vi "RunAsStartupBuzzerTest.vi"() -> ()   [LabVIEW 2020]
uses:
  <vilib>/CISH Robotics/L4VMX VMXpi/Type Def/VMX Channel Index.ctl
  <vilib>/CISH Robotics/L4VMX VMXpi/Digital Output/Digital Output.lvclass
  <vilib>/CISH Robotics/L4VMX VMXpi/L4VMX.lvlib
  <vilib>/CISH Robotics/L4VMX VMXpi/Digital Input/Digital Input.lvclass
panel:
  in  "Stop Button":bool
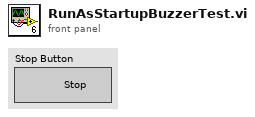
[diagram p1: front panel]
types:
  T1 = typedef "L4VMX.lvlib/VMX Channel Index.ctl" = enum16{"0", "1", "2", "3", "4", "5", "6", "7", "8", "9", "10", "11", "12", "13", "14", "15", "16", "17", "18", "19", "20", "21", "22", "23", "24", "25", "26", "27", "28", "29", "30", "31", "32", "33"}
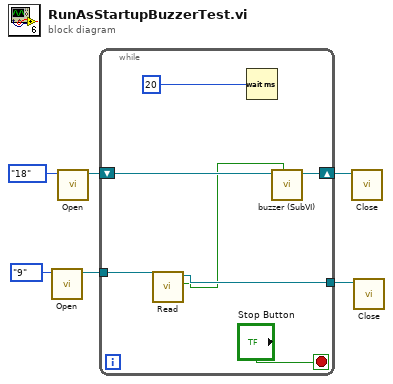
[diagram p0: block diagram]
diagram:
  n1 = call <vilib>:"Open.vi"("VMX Channel Index"=VMX_Channel_Index."9") -> ("Digital Input Object"=w2:refnum<class "Digital Input.lvclass">)  [unwired: 9 in, 1 out]
  n2 = call <vilib>:"Open.vi"("VMX Channel Index"=VMX_Channel_Index."18") -> ("Digital Output Object"=w6:refnum<class "Digital Output.lvclass">)  [unwired: 9 in, 1 out]
  n3 = while {
    shift-right: [w12] -> w5
    shift-left: w6 -> [w13]
    tunnel: w2 -> [w9]
    tunnel: [w8] -> w1
    stop <- "Stop Button" stop-if-true
    n4 = call <vilib>:"Read.vi"("Digital Input Object"=w9) -> ("Value"=w7:bool, "Digital Input Object"=w8:refnum<class "Digital Input.lvclass">)  [unwired: 8 in, 1 out]
    n5 = Wait (ms)(milliseconds to wait=u32 20) -> ()  [unwired: 1 out]
    n6 = call "buzzer (SubVI).vi"("BuzzerOn"=w7, "Digital Output in"=w13) -> ("Digital Output out"=w12:refnum<class "Digital Output.lvclass">)  [unwired: 8 in, 1 out]
  }
  n7 = call <vilib>:"Close.vi"("Digital Output Object"=w5) -> ()  [unwired: 10 in, 1 out]
  n8 = call <vilib>:"Close.vi"("Digital Input Object"=w1) -> ()  [unwired: 10 in, 1 out]
